vi "DAC Configure.vi"(8 "error in":errorcluster, 11 "DAC Shunt dU in":refnum<class "DAC Shunt dU.lvclass">) -> (0 "error out":errorcluster, 3 "DAC Shunt dU out":refnum<class "DAC Shunt dU.lvclass">)   [LabVIEW 2019, in "DAC.lvlib" / "DAC Shunt dU.lvclass"]
uses:
  DAC Shunt dU.lvclass
  DAC.lvclass
  <vilib>/DAQmx/create/channels.llb/DAQmx Create Channel (AI-Voltage-Basic).vi
  C:/Users/krio/Documents/LV_Projects/test-stand/App/DAC/DAC.lvclass
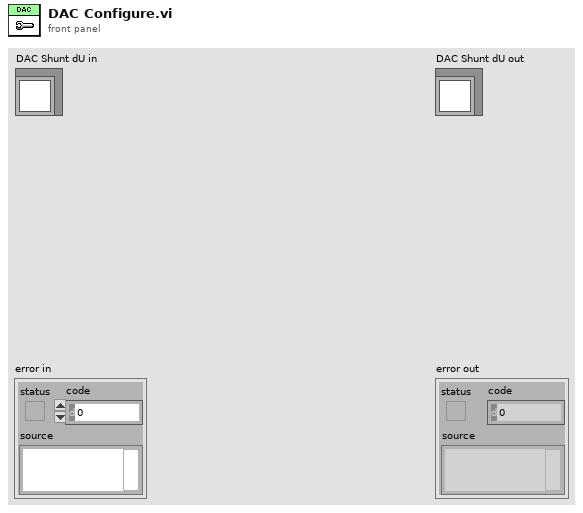
[diagram p1: front panel]
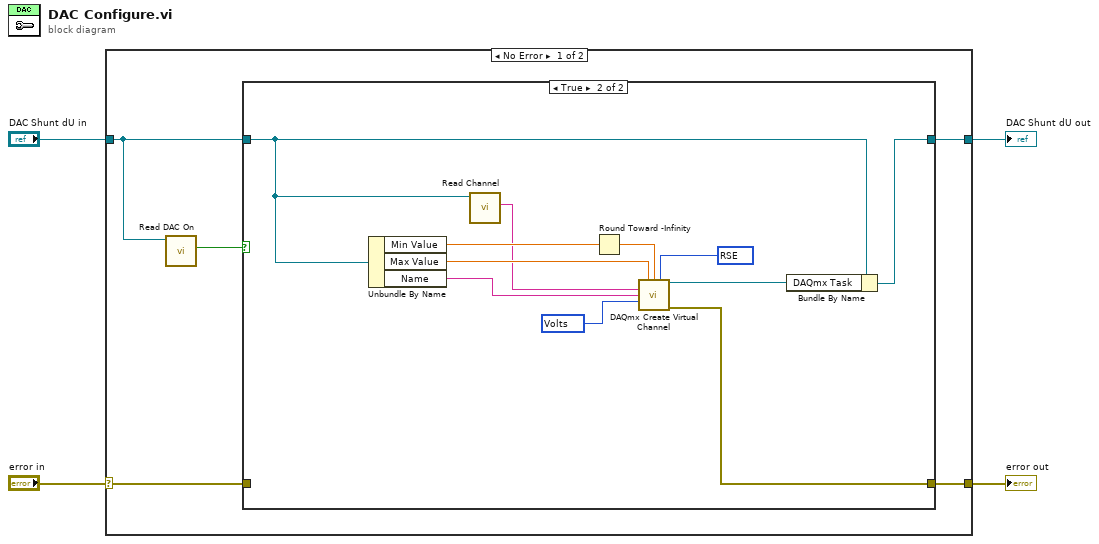
[diagram p0: block diagram]
diagram:
  n1 = case shown="No Error" "error in" {
    selector: "error in" -> [w6 w24]
    tunnel: [w5 w24] -> w4
    tunnel: [w7 w23] -> w3
    tunnel: "DAC Shunt dU in" -> [w9 w23]
    frame No Error {
      n2 = call "Read DAC On.vi"("DAC in"=w9) -> ("DAC On"=w8:bool)  [unwired: 8 in, 2 out]
      n3 = case shown="True" w8 {
        tunnel: w9 -> [w11 w13]
        tunnel: [w11 w21] -> w7
        tunnel: w6 -> [w10 _]
        tunnel: [w10 w19] -> w5
        frame False {
          # "Temperature measurement is off."
        }
        frame True {
          w17 = 10083 items=["Default"=-1, "RSE"=10083, "NRSE"=10078, "Differential"=10106, "Pseudodifferential"=12529] ("input terminal configuration")
          w18 = 10348 items=["Volts"=10348, "From Custom Scale"=10065] ("units")
          # "Temperature measurement is on."
          n4 = Unbundle By Name(w13) -> ("Min Value"=w15:dbl, "Max Value"=w22:dbl, "Name"=w16:string)
          n5 = call "Read Channel.vi"("DAC in"=w13) -> ("Channel"=w12:string)  [unwired: 8 in, 2 out]
          n6 = Round Toward -Infinity(1:w15) -> (0:w14:dbl)
          n7 = call-poly <vilib>:"DAQmx Create Virtual Channel.vi"("maximum value"=w22, "minimum value"=w14, "input terminal configuration"=w17, "physical channels"=w12, "name to assign"=w16, "units"=w18) -> ("task out"=w20:refnum<k21>, "error out"=w19:errorcluster)  [unwired: 8 in]
          n8 = Bundle By Name(cluster=w13, "DAQmx Task"=w20) -> (w21:refnum<class "DAC Shunt dU.lvclass">)
        }
      }
    }
    frame Error {
    }
  }
  "error out" <- w4
  "DAC Shunt dU out" <- w3
